vi "Run.vi"   [LabVIEW 2016]
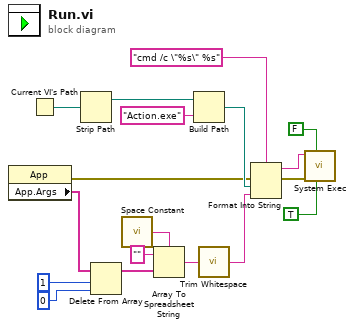
[diagram p0: block diagram]
diagram:
  n1 = property class="App"() -> (error out=w3:errorcluster, "App.Args"=w13:string[])  [unwired: 2 in, 1 out]
  n2 = Current VI's Path() -> (path=w8:path)
  n3 = Strip Path(path=w8) -> (stripped path=w7:path)  [unwired: 1 out]
  n4 = Delete From Array(array=w13, length=1, index=0) -> (array with subset deleted=w12:string[])  [unwired: 1 out]
  n5 = call <vilib>:"Space Constant.vi"() -> ("String"=w17:string)
  n6 = Array To Spreadsheet String(delimiter (Tab)=w17, array=w12, 3:"" ("format string")) -> (spreadsheet string=w14:string)
  n7 = Build Path(base path=w7, name or relative path="Action.exe") -> (appended path=w4:path)
  n8 = call <vilib>:"Trim Whitespace.vi"("string"=w14) -> ("trimmed string"=w2:string)  [unwired: 1 in]
  n9 = Format Into String(format string="cmd /c \"%s\" %s", error in=w3, w4, w2) -> (resulting string=w16:string, error out=w9:errorcluster)  [unwired: 1 in]
  n10 = call <vilib>:"System Exec.vi"("run minimized? (F)"=TRUE, "wait until completion? (T)"=FALSE, "error in (no error)"=w9, "command line"=w16) -> ()  [unwired: 4 in, 4 out]
